vi "Write Data.vi"(8 "error in (no error)":errorcluster, 9 "Publication Time":timestamp, 10 "Value":variant, 11 "TerminalBinding in":refnum<class "TerminalBinding.lvclass">) -> (0 "error out":errorcluster, 3 "TerminalBinding out":refnum<class "TerminalBinding.lvclass">)   [LabVIEW 2015, in "Mediator.lvlib" / "TerminalBinding.lvclass"]
uses:
  TerminalBinding.lvclass
  TerminalBinding.lvclass/TerminalBinding.ctl
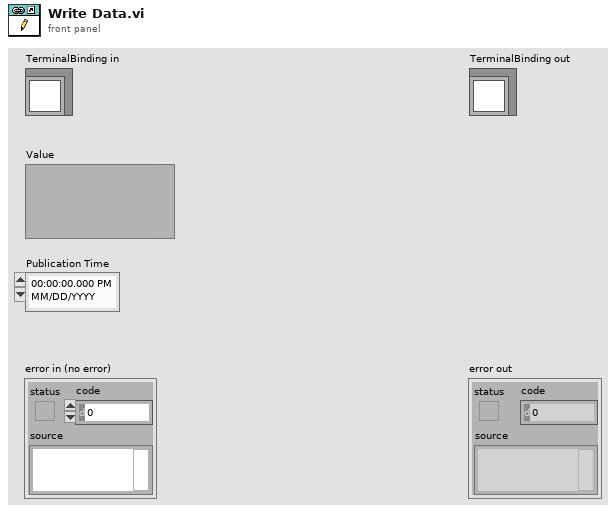
[diagram p1: front panel]
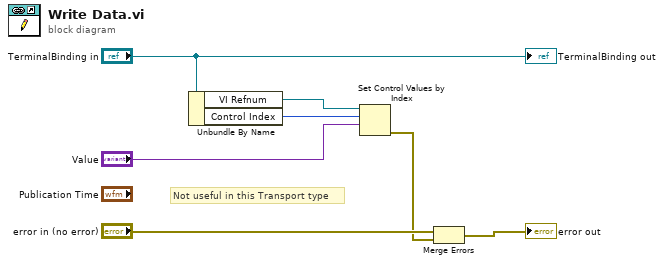
[diagram p0: block diagram]
diagram:
  # "Not useful in this Transport type"
  n1 = Unbundle By Name("TerminalBinding in") -> ("VI Refnum"=w4:refnum<vi>, "Control Index"=w5:i32)
  n2 = Set Control Values by Index(0:w4, 1:w5, 2:"Value") -> (11:w2:errorcluster)  [unwired: 1 in]
  n3 = Merge Errors("error in (no error)", w2) -> (→"error out":errorcluster)
  "TerminalBinding out" <- "TerminalBinding in"
